vi "Test_Parser.vi"() -> ()   [LabVIEW 2018]
uses:
  Classes/STDF File Parser/STDF File Parser.lvclass
  Classes/STDF File Parser/STDF File Parser.lvclass/STDF File Parser.ctl
  <vilib>/Utility/error.llb/Error Cluster From Error Code.vi
panel:
  out "error out":errorcluster
  in  "STDF Files":path[](array[path])
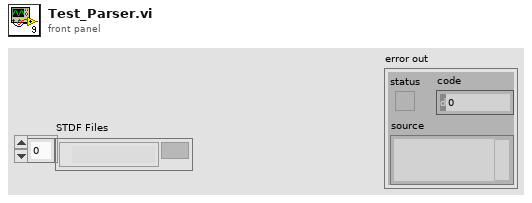
[diagram p1: front panel]
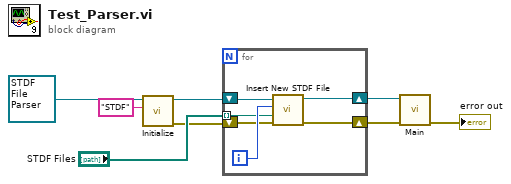
[diagram p0: block diagram]
diagram:
  n1 = call "Initialize.vi"("Parser Name"="STDF", "STDF File Parser in"=refnum<class "STDF File Parser.lvclass"> refnum ("STDF File Parser.lvclass")) -> ("error out"=w4:errorcluster, "STDF File Parser out"=w6:refnum<class "STDF File Parser.lvclass">)  [unwired: 8 in]
  n2 = for {
    tunnel: "STDF Files" -> [w12] mode=indexing
    shift-right: [w11] -> w2
    shift-left: w4 -> [w10]
    shift-right: [w9] -> w3
    shift-left: w6 -> [w14]
    i -> [w13]
    n3 = call "Insert New STDF File.vi"("error in (no error)"=w10, "STDF File"=w12, "Tester #"=w13, "STDF File Parser in"=w14) -> ("error out"=w11:errorcluster, "STDF File Parser out"=w9:refnum<class "STDF File Parser.lvclass">)  [unwired: 6 in]
  }
  n4 = call "Main.vi"("error in (no error)"=w2, "STDF File Parser in"=w3) -> ("error out"=→"error out":errorcluster)  [unwired: 8 in, 1 out]
